vi "Level Detector (Deadtime, Hysteresis).vi"(0 "Data in":dbl[](array[numeric]), 5 "Threshold (V)":dbl, 7 "Hysteresis (V)":dbl, 9 "Deadtime (samples)":i32, 11 "error in":errorcluster) -> (4 "Indices":i32[](array[numeric]), 15 "error out":errorcluster)   [LabVIEW 2015]
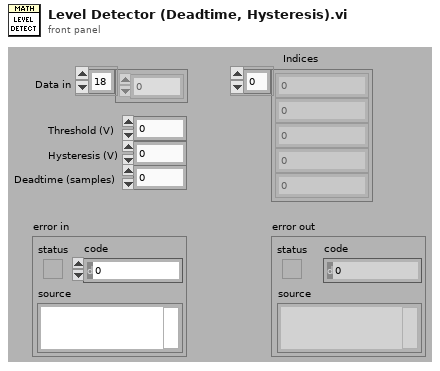
[diagram p1: front panel]
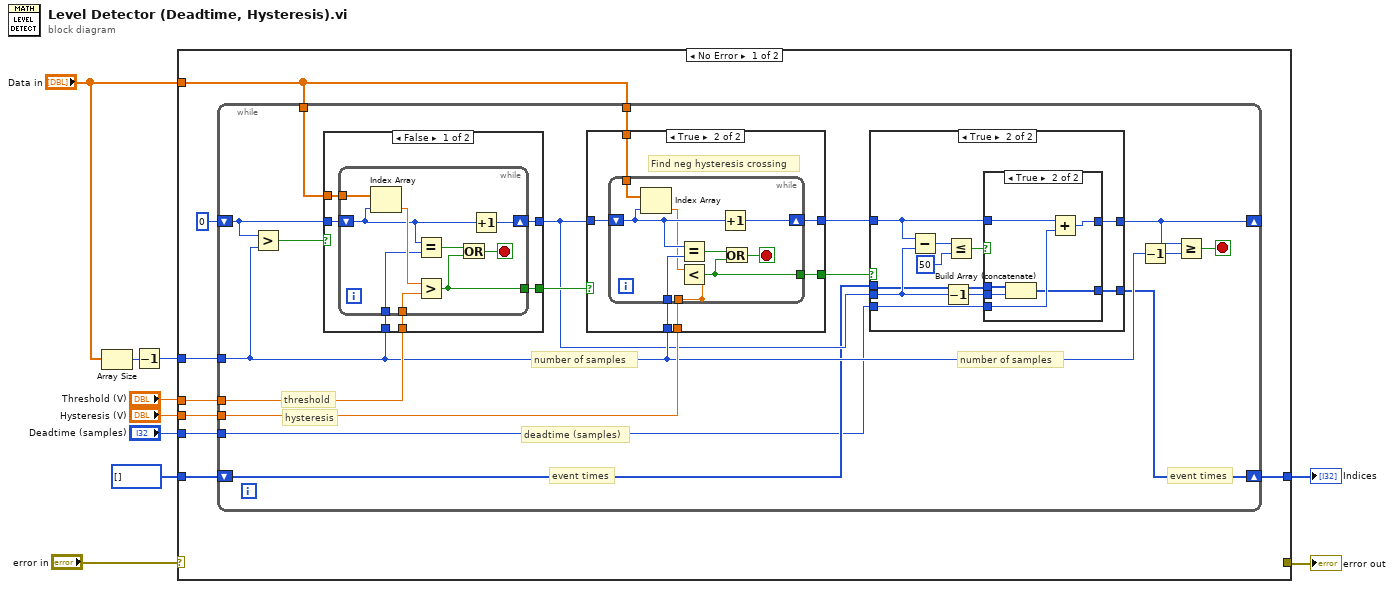
[diagram p0: block diagram]
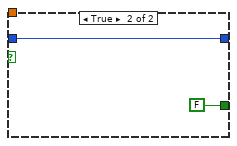
[diagram p4: hidden frame]
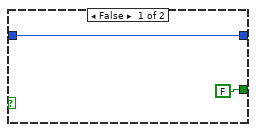
[diagram p5: hidden frame]
diagram:
  n1 = Array Size(array="Data in") -> (size(s)=w9:i32)
  n2 = Decrement(x=w9) -> (x-1=w8:i32)
  n3 = case shown="No Error" "error in" {
    selector: "error in" -> [_ w91]
    tunnel: "Threshold (V)" -> [w18 _]
    tunnel: "Data in" -> [w13 _]
    tunnel: w8 -> [w17 _]
    tunnel: "Deadtime (samples)" -> [w11 _]
    tunnel: [_ w91] -> w6
    tunnel: [w16 w90] -> w4
    tunnel: "Hysteresis (V)" -> [w15 _]
    tunnel: i32[] [] -> [w14 w90]
    frame No Error {
      n4 = while {
        tunnel: w13 -> [w30]
        shift-right: [w25] -> _
        shift-left: 0 ("Index Out") -> [w34]
        tunnel: w18 -> [w31]
        tunnel: w17 -> [w23]
        tunnel: w13 -> [w35]
        shift-right: [w20] -> w16
        shift-left: w14 -> [w21]
        tunnel: w15 -> [w32]
        tunnel: w11 -> [w19]
        stop <- w26 stop-if-true
        # "deadtime (samples)"
        # "event times"
        # "number of samples"
        # "number of samples"
        # "event times"
        # "threshold"
        # "hysteresis"
        n5 = Greater?(x=w34, y=w23) -> (0:w29:bool)
        n6 = case shown="False" w29 {
          tunnel: w30 -> [w61 _]
          tunnel: w34 -> [w60 w72]
          tunnel: [w56 w72] -> w22
          tunnel: w23 -> [w58 _]
          tunnel: w31 -> [w59 _]
          tunnel: [w57 FALSE] -> w28
          frame False {
            n7 = while {
              tunnel: w61 -> [w66]
              shift-right: [w68] -> w56
              shift-left: w60 -> [w65]
              tunnel: w59 -> [w64]
              tunnel: w58 -> [w63]
              tunnel: [w62] -> w57
              stop <- w69 stop-if-true
              n8 = Index Array(array=w66, index=w65) -> (element=w70:dbl)
              n9 = Equal?(x=w65, y=w63) -> (x = y?=w67:bool)
              n10 = Greater?(x=w70, y=w64) -> (0:w62:bool)
              n11 = Or(x=w67, y=w62) -> (x .or. y?=w69:bool)
              n12 = Increment(x=w65) -> (x+1=w68:i32)
            }
          }
          frame True {
          }
        }
        n13 = case shown="True" w28 {
          tunnel: w35 -> [_ w80]
          tunnel: w23 -> [_ w79]
          tunnel: [w74 w78] -> w33
          tunnel: w22 -> [w74 w77]
          tunnel: w32 -> [_ w76]
          tunnel: [FALSE w75] -> w27
          frame False {
          }
          frame True {
            # "Find neg hysteresis crossing"
            n14 = while {
              shift-right: [w88] -> w78
              shift-left: w77 -> [w89]
              tunnel: w79 -> [w87]
              tunnel: w80 -> [w86]
              tunnel: [w82] -> _
              tunnel: w76 -> [w82]
              tunnel: [w81] -> w75
              stop <- w85 stop-if-true
              n15 = Index Array(array=w86, index=w89) -> (element=w83:dbl)
              n16 = Equal?(x=w89, y=w87) -> (x = y?=w84:bool)
              n17 = Less?(x=w83, y=w82) -> (x < y?=w81:bool)
              n18 = Increment(x=w89) -> (x+1=w88:i32)
              n19 = Or(x=w84, y=w81) -> (x .or. y?=w85:bool)
            }
          }
        }
        n20 = case shown="True" w27 {
          tunnel: w19 -> [_ w41]
          tunnel: [w37 w42] -> w25
          tunnel: w33 -> [w37 w43]
          tunnel: w22 -> [_ w44]
          tunnel: w21 -> [w36 w40]
          tunnel: [w36 w39] -> w20
          frame False {
          }
          frame True {
            n21 = Subtract(x=w43, y=w44) -> (x-y=w47:i32)
            n22 = Decrement(x=w44) -> (x-1=w38:i32)
            n23 = Less Or Equal?(x=w47, y=50) -> (x <= y?=w45:bool)
            n24 = case shown="True" w45 {
              tunnel: w38 -> [_ w51]
              tunnel: w43 -> [w49 w54]
              tunnel: [w49 w55] -> w42
              tunnel: w41 -> [_ w53]
              tunnel: w40 -> [w48 w52]
              tunnel: [w48 w50] -> w39
              frame False {
              }
              frame True {
                n25 = Build Array (concatenate)(w52, w51) -> (w50:i32[])
                n26 = Add(x=w54, y=w53) -> (x+y=w55:i32)
              }
            }
          }
        }
        n27 = Decrement(x=w23) -> (x-1=w24:i32)
        n28 = Greater Or Equal?(x=w25, y=w24) -> (x >= y?=w26:bool)
      }
    }
    frame Error {
    }
  }
  "error out" <- w6
  "Indices" <- w4
